vi "Write Nested Viewable Enqueuers.vi"(8 "error in (no error)":errorcluster, 9 "Viewable Labels (optional)":string[](array[string]), 10 "Nested Viewable Enqueuers":refnum<class "Message Enqueuer.lvclass">[](array[class]), 11 "IViewModel In":refnum<class "IViewModel.lvclass">) -> (0 "error out":errorcluster, 3 "IViewModel Out":refnum<class "IViewModel.lvclass">)   [LabVIEW 2020, in "IViewModel.lvlib" / "IViewModel.lvclass"]
doc: "<License>\nCopyright © 2017 Composed Systems, LLC | All rights reserved\nwww.composed.io\n\nAuthor: Ethan Stern <ethan.stern@composed.io>\n\nThis software is provided \"AS IS\" WITHOUT WARRANTIES, either express or implied, AND IS FOR EDUCATIONAL PURPOSES ONLY.\n</License>"
uses:
  <vilib>/gpm_packages/@cs/mva-viewable/Source/IViewModel/IViewModel/IViewModel.lvclass
  <vilib>/ActorFramework/Message Enqueuer/Message Enqueuer.lvclass
  <vilib>/gpm_packages/@cs/mva-viewable/Source/IViewModel/IViewModel/IViewModel.lvclass/IViewModel.ctl
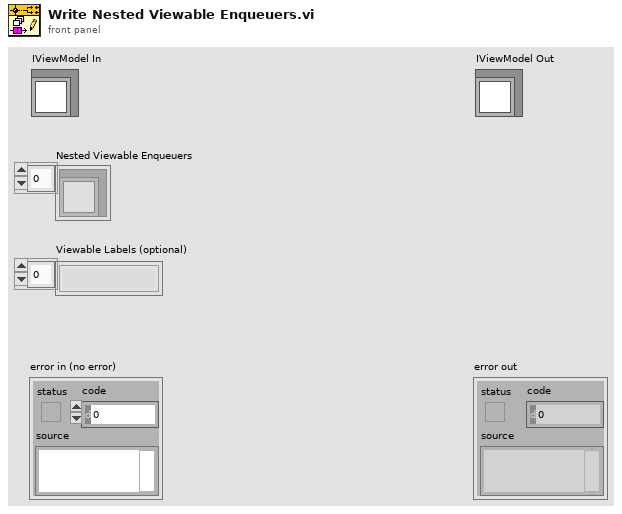
[diagram p1: front panel]
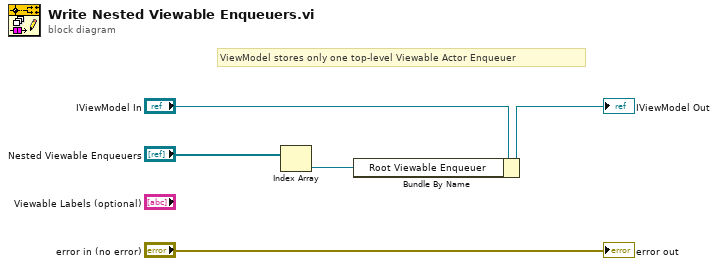
[diagram p0: block diagram]
diagram:
  # "ViewModel stores only one top-level Viewable Actor Enqueuer"
  n1 = Index Array(array="Nested Viewable Enqueuers") -> (element=w2:refnum<class "Message Enqueuer.lvclass">)  [unwired: 1 in]
  n2 = Bundle By Name(cluster="IViewModel In", "Root Viewable Enqueuer"=w2) -> (→"IViewModel Out":refnum<class "IViewModel.lvclass">)
  "error out" <- "error in (no error)"
